vi "Restore (SubVI).vi"(8 "error in (no error)":errorcluster, 11 "Workspace":path=path "C:/Users/1adri/AppData/Local/myDLTS/workspace") -> (0 "error out":errorcluster, 1 "Session properties":T1, 2 "ZIP file path":path, 3 "Workspace path":path, 5 "Canceled":bool)   [LabVIEW 2019]
doc: "Checks for improperly closed files, handles restoration ,displays GUI window"
uses:
  Type defs/Session properties Type Def.ctl
  Type defs/Opened session file index Type Def.ctl
  Type defs/Opened session file info Type Def.ctl
  <vilib>/Utility/sysdir.llb/System Directory Type.ctl
panel:
  in  "Restore":bool
  in  "Remove":bool
  in  "Cancel":bool
  in  "Listbox":i32(listbox)
  # "Some improperly saved files have been detected.\nYou may review these files below and choose whether to restore or permanently delete them."
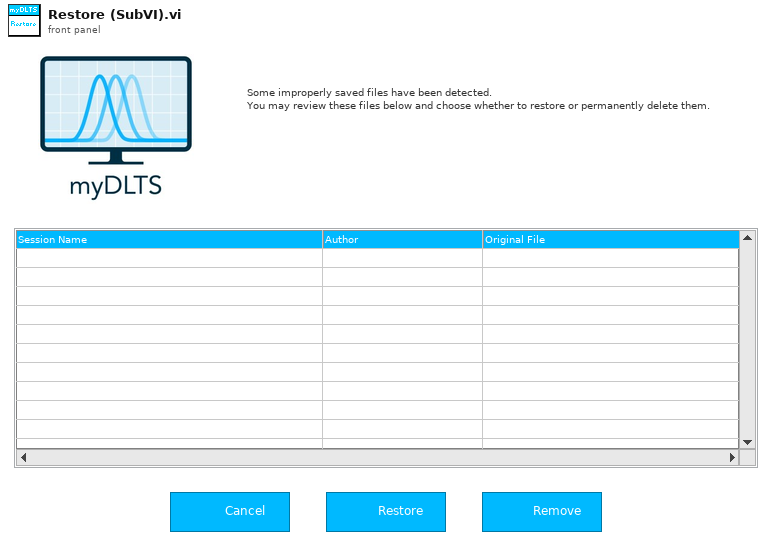
[diagram p1: front panel]
types:
  T1 = typedef "Session properties Type Def.ctl" = cluster{"Session name":string, "Comment":string, "User":string, "Software version":dbl, "Created":timestamp, "Modified":timestamp, "Binary":bool, "GUID":string}
  T2 = typedef "Opened session file index Type Def.ctl" = cluster{"File":T3[]}
  T3 = typedef "Opened session file info Type Def.ctl" = cluster{"Session name":string, "User":string, "ZIP file path":path, "Workspace path":path}
  T4 = enum32{"Invalid", "Standard", "Closed", "Hidden", "Minimized", "Maximized"}
  T5 = typedef "System Directory Type.ctl" = i32
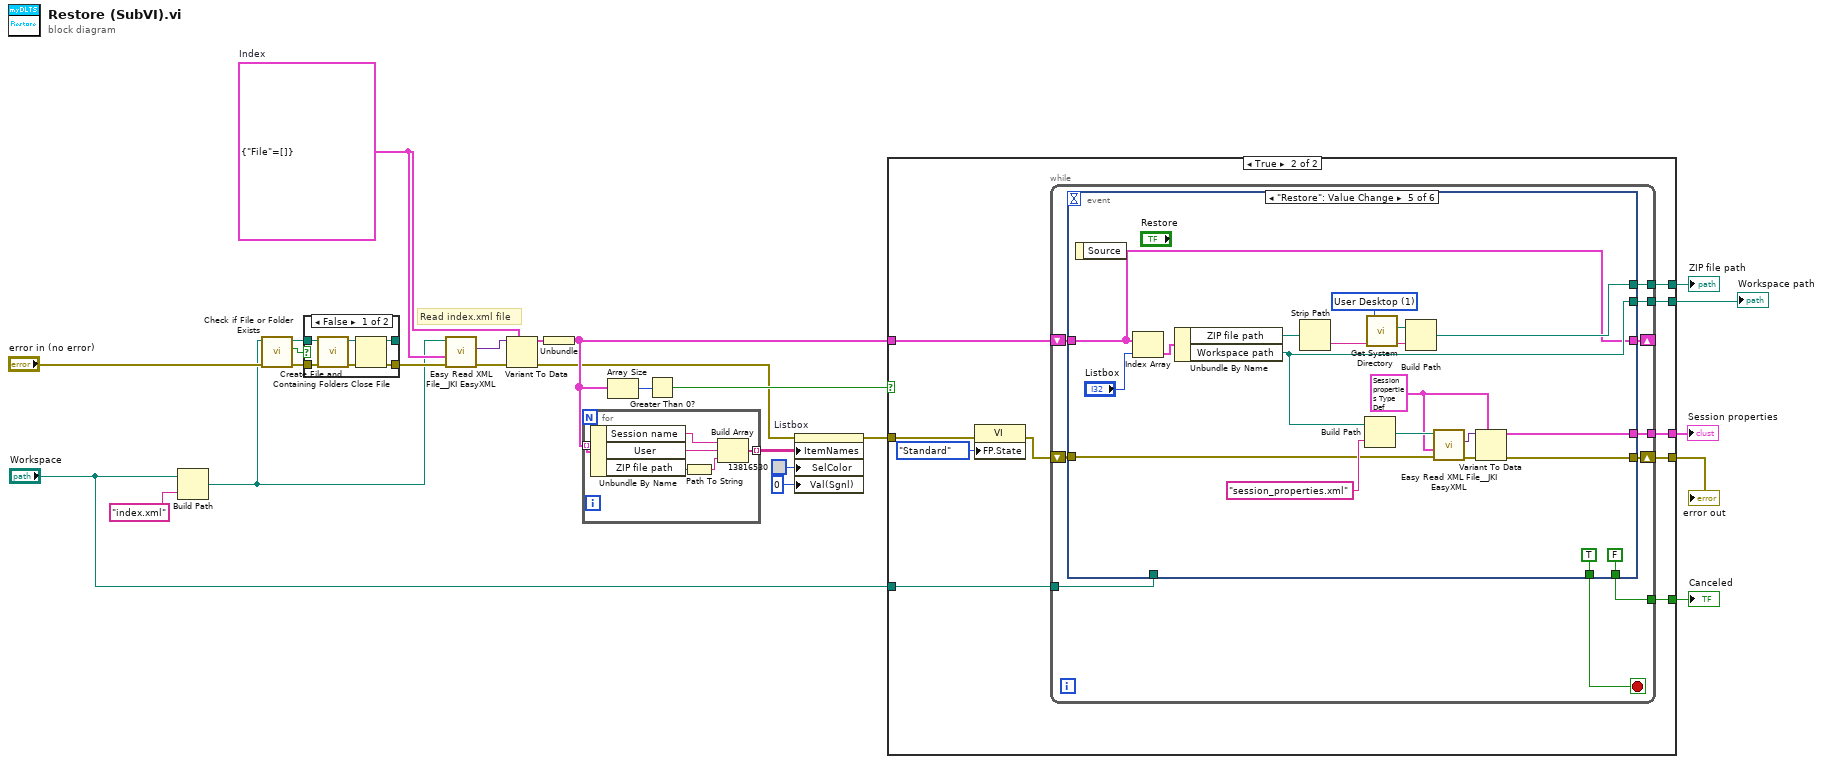
[diagram p0: block diagram]
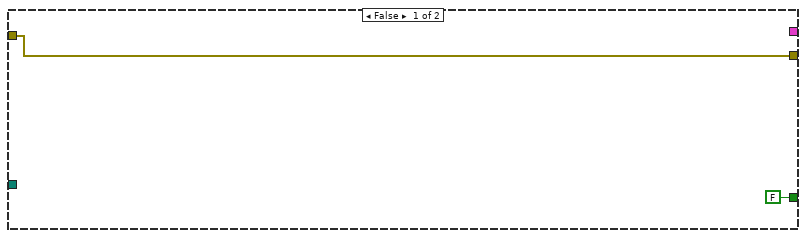
[diagram p2: hidden frame]
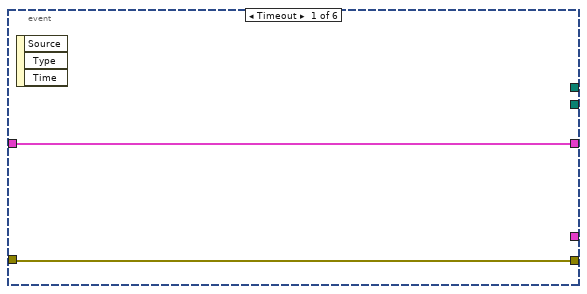
[diagram p3: hidden frame]
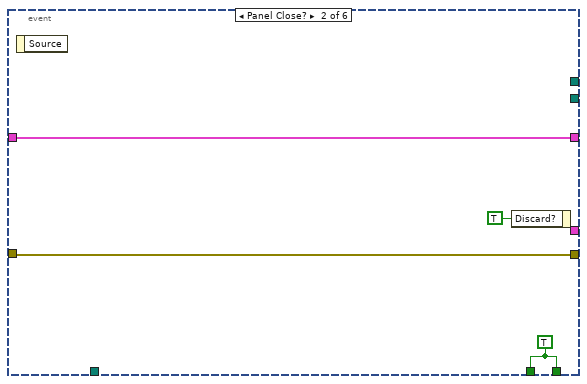
[diagram p4: hidden frame]
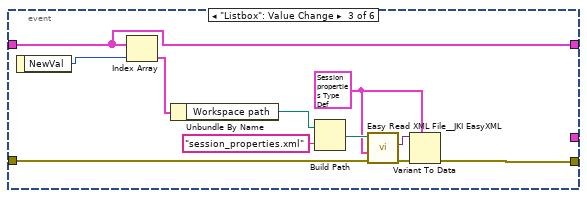
[diagram p5: hidden frame]
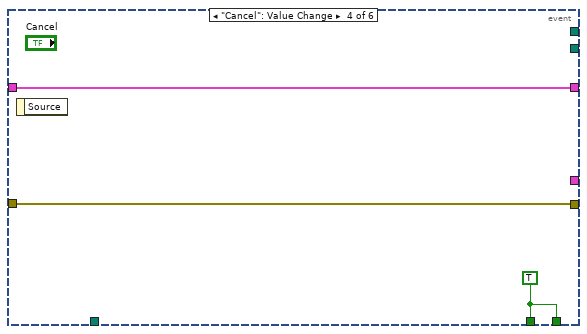
[diagram p6: hidden frame]
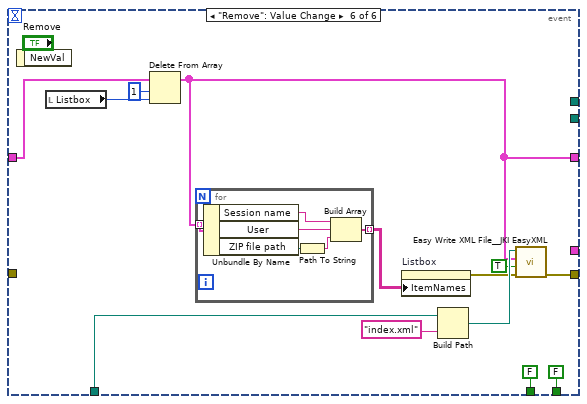
[diagram p7: hidden frame]
diagram:
  w22 = T2 {"File"=[]}  # Index
  # "Read index.xml file"
  n1 = Build Path(base path="Workspace", name or relative path="index.xml") -> (appended path=w8:path)
  n2 = call <vilib>:"Check if File or Folder Exists.vi"("error in (no error)"="error in (no error)", "path"=w8) -> ("error out"=w19:errorcluster, "file or folder exists?"=w18:bool, "dup path"=w20:path)  [unwired: 7 in]
  n3 = case shown="False" w18 {
    tunnel: w20 -> [w29 w32]
    tunnel: w19 -> [w28 w33]
    tunnel: [w27 w33] -> w16
    tunnel: [w26 w32] -> _
    frame False {
      n4 = call <vilib>:"Create File and Containing Folders.vi"("error in (no error)"=w28, "file path"=w29) -> ("error out"=w30:errorcluster, "refnum out"=w31:refnum<file>)  [unwired: 8 in]
      n5 = Close File(refnum=w31, error in=w30) -> (path=w26:path, error out=w27:errorcluster)
    }
    frame True {
    }
  }
  n6 = call <vilib>:"Easy Read XML File__JKI EasyXML.vi"("error in (no error)"=w16, "LabVIEW Data (Type)"=w22, "XML File Path"=w8) -> ("error out"=w25:errorcluster, "LabVIEW Data"=w24:variant)  [unwired: 6 in, 1 out]
  n7 = Variant To Data(error in=w25, type=w22, Variant=w24) -> (data=w23:T2, error out=w10:errorcluster)
  n8 = Unbundle(w23) -> ("File"=w12:T3[])
  n9 = for {
    tunnel: w12 -> [w39] mode=indexing
    tunnel: [w36] -> w11 mode=indexing
    n10 = Unbundle By Name(w39) -> ("Session name"=w38:string, "User"=w37:string, "ZIP file path"=w35:path)
    n11 = Path To String(path=w35) -> (string=w34:string)
    n12 = Build Array(w38, w37, w34) -> (w36:string[])
  }
  n13 = Array Size(array=w12) -> (size(s)=w15:i32)
  n14 = Greater Than 0?(x=w15) -> (x > 0?=w14:bool)
  n15 = property on="Listbox" class="MCListbox (strict)"(error in=w10, "ItemNames"=w11, "SelColor"=u32 13816530 ("Selection Color"), "Val(Sgnl)"=0 ("Value (Signaling)")) -> (error out=w7:errorcluster)  [unwired: 1 in, 1 out]
  n16 = case shown="True" w14 {
    tunnel: w12 -> [_ w48]
    tunnel: w7 -> [w40 w51]
    tunnel: "Workspace" -> [_ w49]
    tunnel: [FALSE w47] -> w5
    tunnel: [_ w46] -> w3
    tunnel: [_ w45] -> w4
    tunnel: [_ w44] -> w2
    tunnel: [w40 w42] -> w1
    frame False {
    }
    frame True {
      n17 = property class="VI"(error in=w51, "FP.State"=T4."Standard" ("Front Panel Window:State")) -> (error out=w43:errorcluster)  [unwired: 1 in, 1 out]
      n18 = while {
        tunnel: w49 -> [w52]
        tunnel: [w59] -> w47
        tunnel: [w58] -> w46
        tunnel: [w57] -> w45
        tunnel: [w56] -> w44
        shift-right: [w54] -> w42
        shift-left: w43 -> [w55]
        shift-right: [w53] -> _
        shift-left: w48 -> [w60]
        stop <- w61 stop-if-true
        n19 = event shown="[4] \"Restore\": Value Change" {
          selector: _ -> [_ _ _ _ _ _]
          dyn-events: _ -> [_ _ _ _ _ _]
          timeout: _ -> [_ _ _ _ _ _]
          tunnel: [_ w66 _ w81 TRUE FALSE] -> w61
          tunnel: w60 -> [w63 w65 w68 w80 w82 w111]
          tunnel: [_ w66 _ w81 FALSE FALSE] -> w59
          tunnel: [_ _ _ _ w93 _] -> w58
          tunnel: [_ _ _ _ w90 _] -> w57
          tunnel: [_ _ _ _ w89 _] -> w56
          tunnel: w55 -> [w62 w64 w69 w79 w88 _]
          tunnel: [w62 w64 w70 w79 w85 w106] -> w54
          tunnel: [w63 w65 w68 w80 w82 w101] -> w53
          tunnel: w52 -> [_ _ _ _ _ w107]
          event Timeout {
            n20 = event-data() -> ()  [unwired: 1 in, 3 out]
          }
          event Panel Close? {
            w66 = TRUE
            n21 = event-data() -> ()  [unwired: 1 in, 1 out]
            n22 = event-data("Discard?"=TRUE) -> ()  [unwired: 1 in, 1 out]
          }
          event "Listbox": Value Change {
            w74 = T1 {"Session name"="", "Comment"="", "User"="", "Software version"=0.0, "Created"=timestamp(0 s since 1904-01-01), "Modified"=timestamp(0 s since 1904-01-01), "Binary"=FALSE, "GUID"=""} ("Session properties")
            n23 = event-data() -> ("NewVal"=w73:i32)  [unwired: 1 in]
            n24 = Index Array(array=w68, index=w73) -> (element=w72:T3)
            n25 = Unbundle By Name(w72) -> ("Workspace path"=w71:path)
            n26 = Build Path(base path=w71, name or relative path="session_properties.xml") -> (appended path=w76:path)
            n27 = call <vilib>:"Easy Read XML File__JKI EasyXML.vi"("error in (no error)"=w69, "LabVIEW Data (Type)"=w74, "XML File Path"=w76) -> ("error out"=w77:errorcluster, "LabVIEW Data"=w78:variant)  [unwired: 6 in, 1 out]
            n28 = Variant To Data(error in=w77, type=w74, Variant=w78) -> (error out=w70:errorcluster)  [unwired: 1 out]
          }
          event "Cancel": Value Change {
            w81 = TRUE
            n29 = event-data() -> ()  [unwired: 1 in, 1 out]
          }
          event "Restore": Value Change {
            w84 = T5 1 items=["User Home"=0, "User Desktop"=1, "User Documents"=2, "User Application Data"=3, "User Preferences"=4, "User Temporary"=5, "Public Documents"=6, "Public Application Data"=7, "Public Preferences"=8, "Public Cache"=13, "System Core Libraries"=9, "System Installed Libraries"=10, "Application Files"=11, "Boot Volume Root"=12] ("system directory type")
            w96 = T1 {"Session name"="", "Comment"="", "User"="", "Software version"=0.0, "Created"=timestamp(0 s since 1904-01-01), "Modified"=timestamp(0 s since 1904-01-01), "Binary"=FALSE, "GUID"=""} ("Session properties")
            n30 = event-data() -> ()  [unwired: 1 in, 1 out]
            n31 = Index Array(array=w82, index="Listbox") -> (element=w95:T3)
            n32 = Unbundle By Name(w95) -> ("ZIP file path"=w92:path, "Workspace path"=w93:path)
            n33 = Strip Path(path=w92) -> (name=w91:string)  [unwired: 1 out]
            n34 = Build Path(base path=w93, name or relative path="session_properties.xml") -> (appended path=w98:path)
            n35 = call <vilib>:"Get System Directory.vi"("system directory type"=w84) -> ("system directory"=w83:path)  [unwired: 10 in]
            n36 = Build Path(base path=w83, name or relative path=w91) -> (appended path=w90:path)
            n37 = call <vilib>:"Easy Read XML File__JKI EasyXML.vi"("error in (no error)"=w88, "LabVIEW Data (Type)"=w96, "XML File Path"=w98) -> ("error out"=w99:errorcluster, "LabVIEW Data"=w100:variant)  [unwired: 6 in, 1 out]
            n38 = Variant To Data(error in=w99, type=w96, Variant=w100) -> (data=w89:T1, error out=w85:errorcluster)
          }
          event "Remove": Value Change {
            n39 = event-data() -> ()  [unwired: 1 in, 1 out]
            n40 = local read "Listbox"() -> (w109:i32)
            n41 = Delete From Array(array=w111, length=1, index=w109) -> (array with subset deleted=w101:T3[])  [unwired: 1 out]
            n42 = for {
              tunnel: w101 -> [w119] mode=indexing
              tunnel: [w116] -> w102 mode=indexing
              n43 = Unbundle By Name(w119) -> ("Session name"=w118:string, "User"=w117:string, "ZIP file path"=w115:path)
              n44 = Path To String(path=w115) -> (string=w114:string)
              n45 = Build Array(w118, w117, w114) -> (w116:string[])
            }
            n46 = property on="Listbox" class="MCListbox (strict)"("ItemNames"=w102) -> (error out=w103:errorcluster)  [unwired: 2 in, 1 out]
            n47 = Build Path(base path=w107, name or relative path="index.xml") -> (appended path=w105:path)
            n48 = call <vilib>:"Easy Write XML File__JKI EasyXML.vi"("error in (no error)"=w103, "Overwrite File? (false)"=TRUE, "LabVIEW Data"=w101, "XML File Path"=w105) -> ("error out"=w106:errorcluster)  [unwired: 6 in, 1 out]
          }
        }
      }
    }
  }
  "Canceled" <- w5
  "ZIP file path" <- w4
  "Workspace path" <- w3
  "Session properties" <- w2
  "error out" <- w1
